vi "Animation.vi"(8 "Error In":errorcluster, 11 "Animation Config":T1) -> (0 "Error Out":errorcluster, 3 "Animation Config":T1)   [LabVIEW 2011, in "LMH-Toolbox.lvlib" / "LMH GUI Tools.lvlib"]
uses:
  LMH GUI Tools.lvlib
  Type Defs/Animation Config.ctl
  <vilib>/picture/picture.llb/imagedata.ctl
  FGVs/Type Defs/Animation FGV State.ctl
  <vilib>/picture/picture.llb/Draw True-Color Pixmap.vi
  LMH-Toolbox.lvlib
panel:
  out "Image":picture
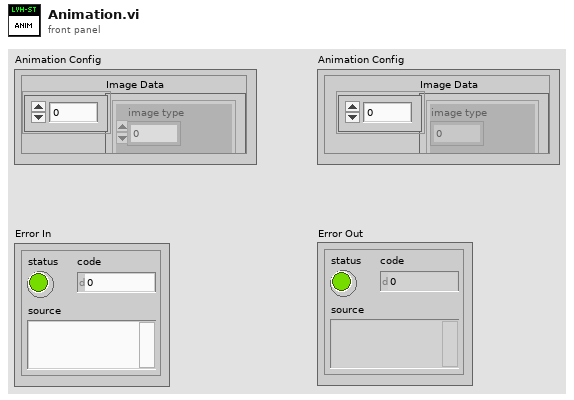
[diagram p1: front panel]
types:
  T1 = typedef "LMH-Toolbox.lvlib/LMH GUI Tools.lvlib/Animation Config.ctl" = cluster{"Image Data":T2[], "Animation Picture Indicator":refnum<vi>, "FPS":u32, "Position":cluster{"X":i16, "Y":i16}}
  T2 = typedef "imagedata.ctl" = cluster{"image type":i32, "image depth":i32, "image":u8[], "mask":u8[], "colors":u32[], "Rectangle":cluster{"left":i16, "top":i16, "right":i16, "bottom":i16}}
  T3 = typedef "LMH-Toolbox.lvlib/LMH GUI Tools.lvlib/Animation FGV State.ctl" = enum16{"Init", "Set", "Get"}
  T4 = enum32{"Invalid", "Standard", "Closed", "Hidden", "Minimized", "Maximized"}
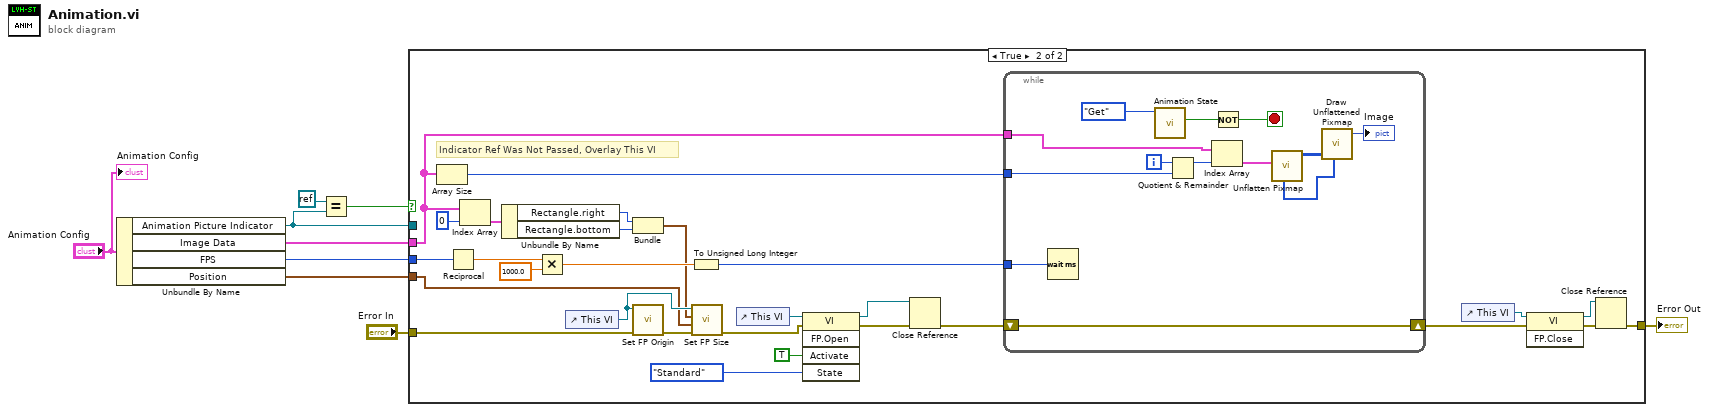
[diagram p0: block diagram]
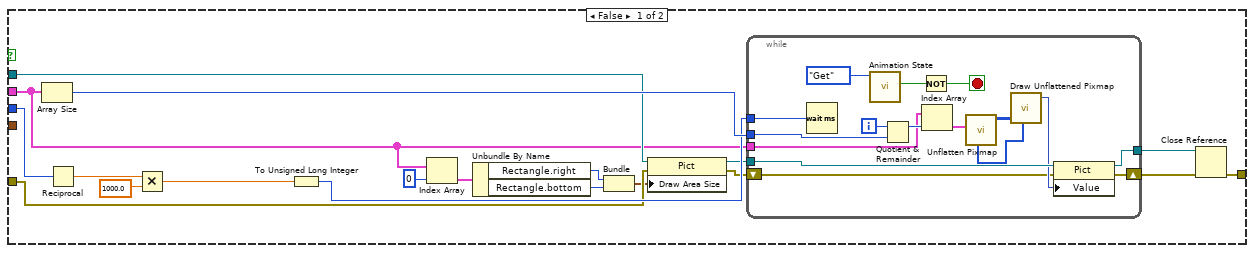
[diagram p2: hidden frame]
diagram:
  n1 = Unbundle By Name("Animation Config") -> ("Animation Picture Indicator"=w2:refnum<vi>, "Image Data"=w8:T2[], "FPS"=w7:u32, "Position"=w6:cluster{"X":i16, "Y":i16})
  n2 = Equal?(x=refnum<k0> refnum, y=w2) -> (x = y?=w4:bool)
  n3 = case shown="True" w4 {
    tunnel: w8 -> [w13 w70]
    tunnel: w7 -> [w20 w65]
    tunnel: [w10 w55] -> w1
    tunnel: w6 -> [_ w53]
    tunnel: "Error In" -> [w18 w52]
    tunnel: w2 -> [w19 _]
    frame False {
      n4 = Array Size(array=w13) -> (size(s)=w28:i32)
      n5 = Reciprocal(x=w20) -> (1/x=w26:dbl)
      n6 = Multiply(x=w26, y=1000.0) -> (x*y=w24:dbl)
      n7 = To Unsigned Long Integer(number=w24) -> (unsigned 32bit integer=w23:u32)
      n8 = Index Array(array=w13, index=0) -> (element=w17:T2)
      n9 = Unbundle By Name(w17) -> ("Rectangle.right"=w22:i16, "Rectangle.bottom"=w21:i16)
      n10 = Bundle("right"=w22, "bottom"=w21) -> (w16:cluster{"right":i16, "bottom":i16})  [unwired: 1 in]
      n11 = property class="Pict"(reference=w19, error in=w18, "Draw Area Size"=w16) -> (reference out=w14:refnum<vi>, error out=w15:errorcluster)
      n12 = while {
        tunnel: w28 -> [w43]
        shift-right: [w32] -> w11
        shift-left: w15 -> [w33]
        tunnel: w23 -> [w36]
        tunnel: w14 -> [w35]
        tunnel: [w31] -> w12
        tunnel: w13 -> [w30]
        i -> [w44]
        stop <- w37 stop-if-true
        n13 = Wait (ms)(milliseconds to wait=w36) -> ()  [unwired: 1 out]
        n14 = call "Animation State.vi"("Function"=Animation_FGV_State."Get") -> ("Running?"=w38:bool)  [unwired: 10 in]
        n15 = Quotient & Remainder(x=w44, y=w43) -> (x-y*floor(x/y)=w42:i32)  [unwired: 1 out]
        n16 = Not(x=w38) -> (.not. x?=w37:bool)
        n17 = Index Array(array=w30, index=w42) -> (element=w29:T2)
        n18 = call <vilib>:"Unflatten Pixmap.vi"("image data"=w29) -> ("24-bit pixmap"=w41:u32[][], "mask"=w40:u8[])  [unwired: 4 in, 5 out]
        n19 = call-poly <vilib>:"Draw Unflattened Pixmap.vi"("data (RGB format)"=w41, "mask"=w40) -> ("new picture"=w34:picture)  [unwired: 7 in]
        n20 = property class="Pict"(reference=w35, error in=w33, "Value"=w34) -> (reference out=w31:refnum<vi>, error out=w32:errorcluster)
      }
      n21 = Close Reference(reference=w12, error in (no error)=w11) -> (error out=w10:errorcluster)
    }
    frame True {
      # "Indicator Ref Was Not Passed, Overlay This VI"
      n22 = Array Size(array=w70) -> (size(s)=w72:i32)
      n23 = Reciprocal(x=w65) -> (1/x=w68:dbl)
      n24 = Index Array(array=w70, index=0) -> (element=w69:T2)
      n25 = Unbundle By Name(w69) -> ("Rectangle.right"=w61:i16, "Rectangle.bottom"=w60:i16)
      n26 = Multiply(x=w68, y=1000.0) -> (x*y=w66:dbl)
      n27 = control-ref of="This VI"() -> (w63:refnum<vi>)
      n28 = Bundle("right"=w61, "bottom"=w60) -> (w59:cluster{"right":i16, "bottom":i16})  [unwired: 1 in]
      n29 = call "Set FP Origin.vi"("Error In"=w52, "VI Ref"=w63) -> ("Error Out"=w62:errorcluster)  [unwired: 9 in]
      n30 = To Unsigned Long Integer(number=w66) -> (unsigned 32bit integer=w64:u32)
      n31 = call "Set FP Size.vi"("Error In"=w62, "Position"=w53, "Size"=w59, "VI Ref"=w63) -> ("Error Out"=w48:errorcluster)  [unwired: 7 in]
      n32 = control-ref of="This VI"() -> (w49:refnum<vi>)
      n33 = invoke class="VI" method="FP.Open"(reference=w49, error in=w48, "Activate"=TRUE ("Activate?"), "State"=T4."Standard") -> (reference out=w50:refnum<vi>, error out=w51:errorcluster)  [unwired: 1 in, 3 out]
      n34 = Close Reference(reference=w50, error in (no error)=w51) -> (error out=w47:errorcluster)
      n35 = while {
        tunnel: w72 -> [w84]
        tunnel: w70 -> [w79]
        shift-right: [w77] -> w54
        shift-left: w47 -> [w77]
        tunnel: w64 -> [w73]
        i -> [w85]
        stop <- w74 stop-if-true
        n36 = Wait (ms)(milliseconds to wait=w73) -> ()  [unwired: 1 out]
        n37 = call "Animation State.vi"("Function"=Animation_FGV_State."Get") -> ("Running?"=w75:bool)  [unwired: 10 in]
        n38 = Quotient & Remainder(x=w85, y=w84) -> (x-y*floor(x/y)=w83:i32)  [unwired: 1 out]
        n39 = Index Array(array=w79, index=w83) -> (element=w78:T2)
        n40 = Not(x=w75) -> (.not. x?=w74:bool)
        n41 = call <vilib>:"Unflatten Pixmap.vi"("image data"=w78) -> ("24-bit pixmap"=w81:u32[][], "mask"=w80:u8[])  [unwired: 4 in, 5 out]
        n42 = call-poly <vilib>:"Draw Unflattened Pixmap.vi"("data (RGB format)"=w81, "mask"=w80) -> ("new picture"=→"Image":picture)  [unwired: 7 in]
      }
      n43 = control-ref of="This VI"() -> (w58:refnum<vi>)
      n44 = invoke class="VI" method="FP.Close"(reference=w58, error in=w54) -> (reference out=w57:refnum<vi>, error out=w56:errorcluster)  [unwired: 1 in, 1 out]
      n45 = Close Reference(reference=w57, error in (no error)=w56) -> (error out=w55:errorcluster)
    }
  }
  "Error Out" <- w1
  "Animation Config" <- "Animation Config"
